vi "Nov15_initialdesign.vi"() -> ()   [LabVIEW 2017]
panel:
  out "Numeric":dbl
  out "Boolean":bool
  out "Numeric 4":dbl
  in  "?":dbl(knob) scale=-10.0..10.0
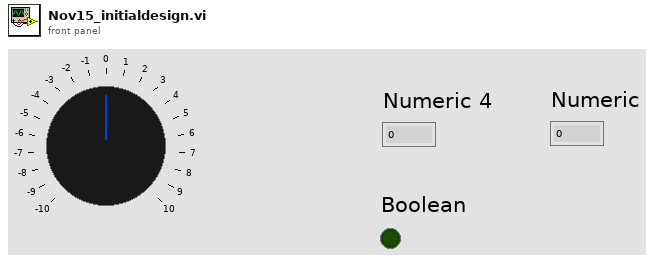
[diagram p1: front panel]
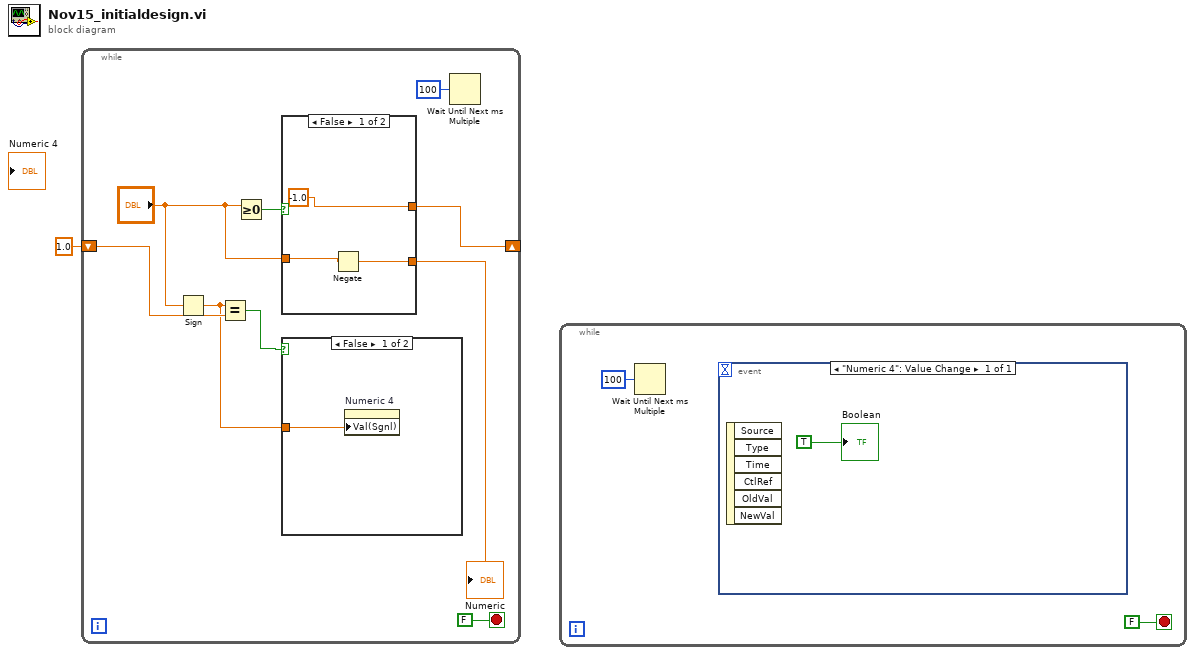
[diagram p0: block diagram]
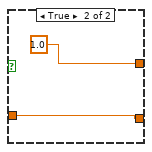
[diagram p3: hidden frame]
diagram:
  n1 = while {
    shift-right: [w7] -> _
    shift-left: 1.0 -> [w5]
    stop <- FALSE stop-if-true
    n2 = Sign(1:"?") -> (0:w3:dbl)
    n3 = Equal?(x=w3, y=w5) -> (x = y?=w4:bool)
    n4 = Greater Or Equal To 0?(x="?") -> (x >= 0?=w10:bool)
    n5 = case shown="False" w10 {
      tunnel: "?" -> [w14 w16]
      tunnel: [w13 w16] -> w2
      tunnel: [-1.0 1.0] -> w7
      frame False {
        n6 = Negate(x=w14) -> (-x=w13:dbl)
      }
      frame True {
      }
    }
    "Numeric" <- w2
    n7 = case shown="False" w4 {
      tunnel: w3 -> [w11 _]
      frame False {
        n8 = property on="Numeric 4" class="DigNum (strict)"("Val(Sgnl)"=w11) -> ()  [unwired: 2 in, 2 out]
      }
      frame True {
      }
    }
    n9 = Wait Until Next ms Multiple(millisecond multiple=u32 100) -> ()  [unwired: 1 out]
  }
  n10 = while {
    stop <- FALSE stop-if-true
    n11 = Wait Until Next ms Multiple(millisecond multiple=u32 100) -> ()  [unwired: 1 out]
    n12 = event shown="[0] \"Numeric 4\": Value Change" {
      selector: _ -> [_]
      dyn-events: _ -> [_]
      timeout: _ -> [_]
      event "Numeric 4": Value Change {
        n13 = event-data() -> ()  [unwired: 1 in, 6 out]
        "Boolean" <- TRUE
      }
    }
  }
